vi "ICM Initializers Path.vi"(8 "error in (no error)":errorcluster) -> (0 "error out":errorcluster, 3 "ICM Queries Path":path)   [LabVIEW 2018]
doc: "ICM Queries Path.vi\n\nThis VI defines where the ICM Queries directory is located.\n\nInstrument Communication Module Version 1.0\nSeptember, 2017 Original Code Consulting David Thomson\n www.originalcode.com"
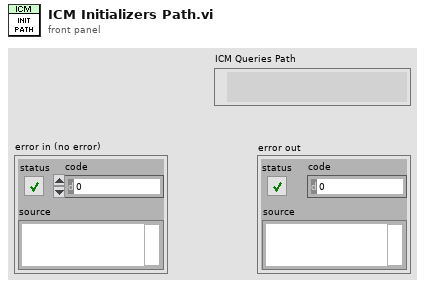
[diagram p1: front panel]
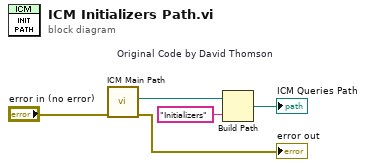
[diagram p0: block diagram]
diagram:
  w4 = "Initializers"  # Original Code by David Thomson
  n1 = call "ICM Main Path.vi"("error in (no error)"="error in (no error)") -> ("error out"=→"error out":errorcluster, "ICM Source Directory"=w2:path)  [unwired: 8 in, 1 out]
  n2 = Build Path(base path=w2, name or relative path=w4) -> (appended path=→"ICM Queries Path":path)
